vi "Window-Exit window.vi"(8 "error in (no error)":errorcluster) -> (0 "error out":errorcluster, 1 "Cancelled (Left button pressed)":bool)   [LabVIEW 2013]
doc: "Use this template to create a dialog box with event handling."
uses:
  <vilib>/Utility/miscctls.llb/LVPointTypeDef.ctl
  Global Variables/General Globals.vi
panel:
  in  "Info":bool
  out "Mesage 2":string="Are you sure you want to stop imaging and shut down the microscope control software?\n(Remember to remove recent data from the local drive)"
  out "Mesage 1":string="Are you sure you want to shut down\nthe microscope control software?"
  in  "Website":bool
  in  "Left Button":bool
  in  "Right button":bool
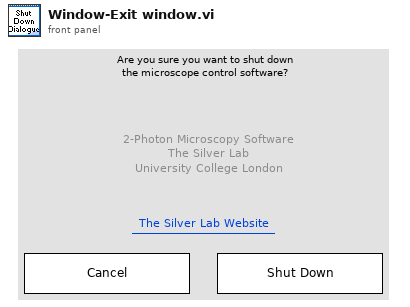
[diagram p1: front panel]
types:
  T1 = typedef "LVPointTypeDef.ctl" = cluster{"Horizontal":i16, "Vertical":i16}
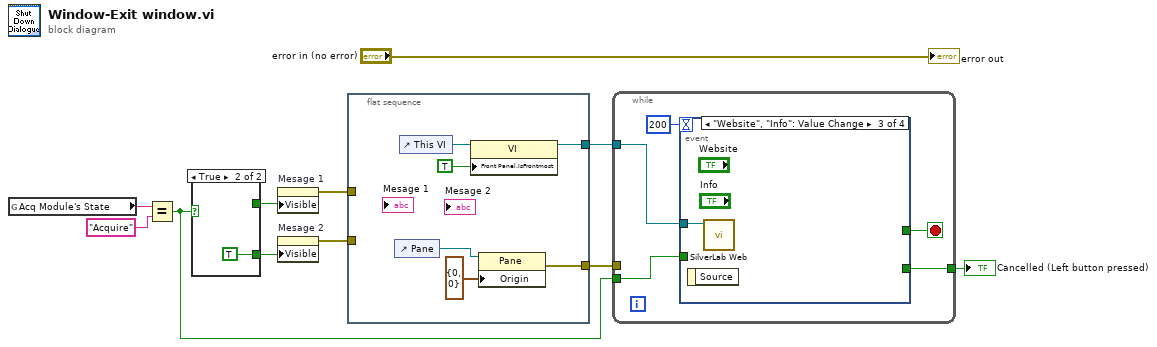
[diagram p0: block diagram]
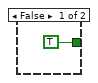
[diagram p2: hidden frame]
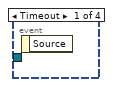
[diagram p3: hidden frame]
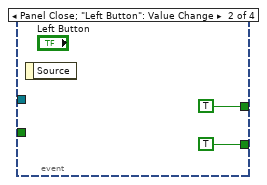
[diagram p4: hidden frame]
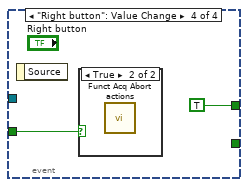
[diagram p5: hidden frame]
diagram:
  n1 = global read "General Globals.vi" "Acq Module's State"() -> (w8:string)
  n2 = Equal?(x=w8, y="Acquire") -> (x = y?=w6:bool)
  n3 = case shown="True" w6 {
    tunnel: [_ TRUE] -> w5
    tunnel: [TRUE _] -> w4
    frame False {
    }
    frame True {
    }
  }
  n4 = property on="Mesage 1" class="Str"("Visible"=w4) -> (error out=w3:errorcluster)  [unwired: 2 in, 1 out]
  n5 = property on="Mesage 2" class="Str"("Visible"=w5) -> (error out=w2:errorcluster)  [unwired: 2 in, 1 out]
  n6 = flat-sequence {
    tunnel: [w16] -> w11
    tunnel: w3 -> [_]
    tunnel: w2 -> [_]
    tunnel: [w14] -> w1
    frame #0 {
      n7 = control-ref of="Pane"() -> (w15:refnum<vi>)
      n8 = control-ref of="This VI"() -> (w18:refnum<vi>)
      n9 = property on="Property Node" class="VI"(reference=w18, "Front Panel.IsFrontmost"=TRUE ("Front Panel Window:Is Frontmost")) -> (reference out=w14:refnum<vi>)  [unwired: 1 in, 1 out]
      n10 = property class="Pane"(reference=w15, "Origin"=T1 {"Horizontal"=0, "Vertical"=0}) -> (error out=w16:errorcluster)  [unwired: 1 in, 1 out]
    }
  }
  n11 = while {
    tunnel: w11 -> [_]
    tunnel: [w22] -> w10
    tunnel: w6 -> [w21]
    tunnel: w1 -> [w20]
    stop <- w24 stop-if-true
    n12 = event shown="[2] \"Website\", \"Info\": Value Change" {
      selector: _ -> [_ _ _ _]
      dyn-events: _ -> [_ _ _ _]
      timeout: 200 -> [_ _ _ _]
      tunnel: [_ TRUE ("Stop?") _ TRUE ("Stop?")] -> w24
      tunnel: [_ TRUE ("Stop subpanel") _ _] -> w22
      tunnel: w21 -> [_ _ _ w28]
      tunnel: w20 -> [_ _ w27 _]
      event Timeout {
        n13 = event-data() -> ()  [unwired: 1 in, 1 out]
      }
      event Panel Close; "Left Button": Value Change {
        n14 = event-data() -> ()  [unwired: 1 in, 1 out]
      }
      event "Website", "Info": Value Change {
        n15 = event-data() -> ()  [unwired: 1 in, 1 out]
        n16 = call "SilverLab Web.vi"("Calle window's ref"=w27) -> ()  [unwired: 11 in]
      }
      event "Right button": Value Change {
        n17 = event-data() -> ()  [unwired: 1 in, 1 out]
        n18 = case shown="True" w28 {
          frame False {
          }
          frame True {
            n19 = call "Funct Acq Abort actions.vi"() -> ()  [unwired: 11 in, 1 out]
          }
        }
      }
    }
  }
  "Cancelled (Left button pressed)" <- w10
  "error out" <- "error in (no error)"
